vi "Handle Pos and Rot.vi"(4 "Starting Line Y":dbl format="%#_13g", 5 "Mouse Up":bool, 6 "Delta":bool, 7 "Picture in":refnum<vi>, 8 "Option":T1, 9 "Coord (ft)":cluster{dbl, dbl}, 10 "Index":i32, 11 "Points in":cluster{"x":dbl, "y":dbl, "th":dbl}[](array[cluster])) -> (3 "Points out":cluster{"x":dbl, "y":dbl, "th":dbl}[](array[cluster]))   [LabVIEW 2023]
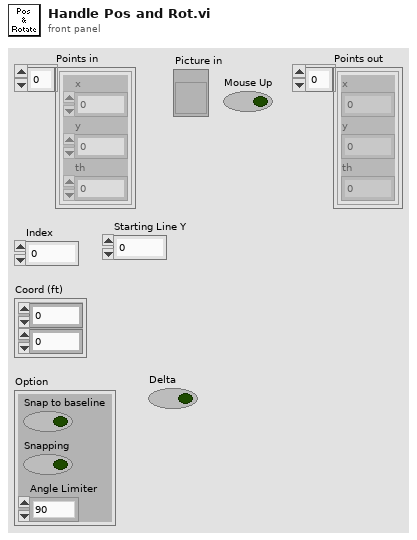
[diagram p1: front panel]
types:
  T1 = cluster{"Snap to baseline":bool, "Snapping":bool, "Angle Limiter":enum16{"90", "45", "15", "1"}}
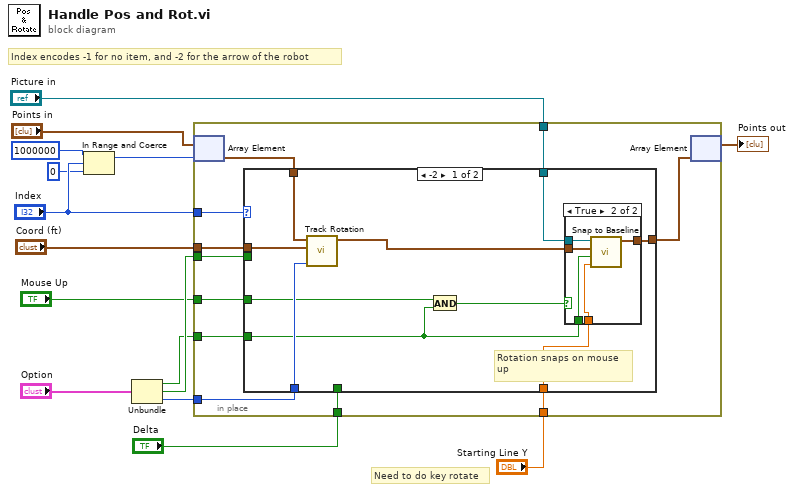
[diagram p0: block diagram]
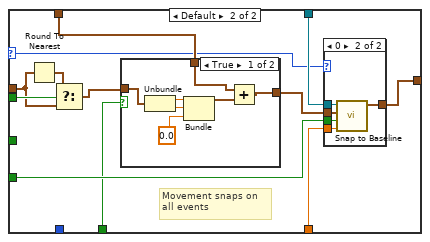
[diagram p3: hidden frame]
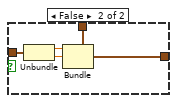
[diagram p4: hidden frame]
diagram:
  # "Need to do key rotate"
  # "Index encodes -1 for no item, and -2 for the arrow of the robot"
  n1 = In Range and Coerce(upper limit=1000000 ("lower limit"), x="Index", lower limit=0) -> (coerced(x)=w3:i32)  [unwired: 1 out]
  n2 = Unbundle("Option") -> ("Snap to baseline"=w13:bool, "Snapping"=w14:bool, "Angle Limiter"=w15:enum16{"90", "45", "15", "1"})
  n3 = in-place {
    in-place-border: "Coord (ft)" -> [w26]
    in-place-border: "Index" -> [w23]
    in-place-border: w14 -> [w22]
    in-place-border: w13 -> [w20]
    in-place-border: w15 -> [w21]
    in-place-border: "Picture in" -> [w19]
    in-place-border: "Mouse Up" -> [w18]
    in-place-border: "Delta" -> [w17]
    in-place-border: "Starting Line Y" -> [w16]
    n4 = in-place-array #1("Points in", w3) -> (w25:cluster{"x":dbl, "y":dbl, "th":dbl})
    n5 = case shown="-2" w23 {
      selector: w23 -> [_ w45]
      tunnel: w26 -> [w36 w52]
      tunnel: w25 -> [w28 w47]
      tunnel: [w29 w46] -> w24
      tunnel: w21 -> [w35 _]
      tunnel: w22 -> [_ w54]
      tunnel: w20 -> [w31 w50]
      tunnel: w19 -> [w34 w48]
      tunnel: w18 -> [w33 _]
      tunnel: w17 -> [_ w44]
      tunnel: w16 -> [w27 w43]
      frame -2 {
        # "Rotation snaps on mouse\nup"
        n6 = call "Track Rotation.vi"("Angle Limiter"=w35, "Coord"=w36, "Point in"=w28) -> ("Point out"=w30:cluster{"x":dbl, "y":dbl, "th":dbl})  [unwired: 8 in]
        n7 = And(x=w33, y=w31) -> (x .and. y?=w32:bool)
        n8 = case shown="True" w32 {
          tunnel: w30 -> [w37 w40]
          tunnel: [w37 w42] -> w29
          tunnel: w34 -> [_ w41]
          tunnel: w31 -> [_ w39]
          tunnel: w27 -> [_ w38]
          frame False {
          }
          frame True {
            n9 = call "Snap to Baseline.vi"("Starting Line Y"=w38, "Snap to baseline"=w39, "Point in"=w40, "Picture in"=w41) -> ("Point out"=w42:cluster{"x":dbl, "y":dbl, "th":dbl})  [unwired: 7 in]
          }
        }
      }
      frame Default {
        # "Movement snaps on\nall events"
        n10 = Round To Nearest(number=w52) -> (nearest integer value=w53:cluster{dbl, dbl})
        n11 = Select(t=w53, s=w54, f=w52) -> (s? t:f=w51:cluster{dbl, dbl})
        n12 = case shown="True" w44 {
          tunnel: w51 -> [w61 w64]
          tunnel: [w57 w63] -> w49
          tunnel: w47 -> [w55 w62]
          frame True {
            n13 = Unbundle(w61) -> (w60:dbl, w59:dbl)
            n14 = Bundle(w60, w59, 0.0) -> (w56:cluster{dbl, dbl, dbl})  [unwired: 1 in]
            n15 = Add(x=w55, y=w56) -> (x+y=w57:cluster{dbl, dbl, dbl})
          }
          frame False {
            n16 = Unbundle(w64) -> (w66:dbl, w65:dbl)
            n17 = Bundle(cluster=w62, "x"=w66, "y"=w65) -> (w63:cluster{"x":dbl, "y":dbl, "th":dbl})  [unwired: 1 in]
          }
        }
        n18 = case shown="0" w45 {
          tunnel: w50 -> [_ w72]
          tunnel: w49 -> [w67 w71]
          tunnel: w48 -> [_ w70]
          tunnel: [w67 w69] -> w46
          tunnel: w43 -> [_ w68]
          frame Default {
          }
          frame 0 {
            n19 = call "Snap to Baseline.vi"("Starting Line Y"=w68, "Snap to baseline"=w72, "Point in"=w71, "Picture in"=w70) -> ("Point out"=w69:cluster{"x":dbl, "y":dbl, "th":dbl})  [unwired: 7 in]
          }
        }
      }
    }
    n20 = in-place-array #1(w24) -> (→"Points out":cluster{"x":dbl, "y":dbl, "th":dbl}[])  [unwired: 1 out]
  }
